vi "Last Ack.vi"(7 "Sender":refnum<class "Sender.lvclass">, 10 "Actor":refnum<class "Actor.lvclass">, 11 "jettl Actor in":refnum<class "jettl Actor.lvclass">) -> (3 "jettl Actor out":refnum<class "jettl Actor.lvclass">)   [LabVIEW 2021, in "jettl.lvlib" / "Temporary Actor.lvlib" / "jettl Actor.lvclass"]
uses:
  jettl Actor.lvclass
  Actor/Actor.lvclass
  Sender/Sender/Sender.lvclass
  jettl Actor.lvclass/jettl Actor.ctl
  Addresses Strategy/Addresses Strategy/Addresses Strategy.lvclass
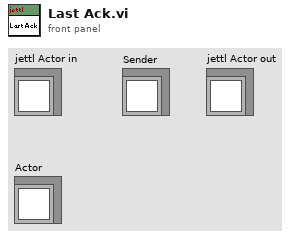
[diagram p1: front panel]
types:
  T1 = typedef "jettl.lvlib/Relation.ctl" = enum16{"Self", "Creator", "Created"}
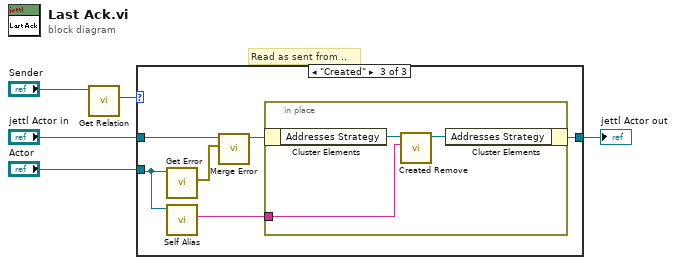
[diagram p0: block diagram]
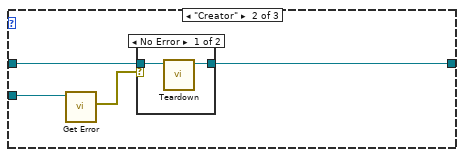
[diagram p3: hidden frame]
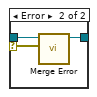
[diagram p4: hidden frame]
diagram:
  # "Read as sent from .."
  n1 = call-dynamic "Get Relation.vi"("Sender in"="Sender") -> ("Relation"=w1:T1)  [unwired: 10 in]
  n2 = case shown="\"Created\"" w1 {
    tunnel: "jettl Actor in" -> [w6 w9 w18]
    tunnel: [w6 w8 w17] -> w4
    tunnel: "Actor" -> [_ w7 w16]
    frame "Self" {
      # "Case will not fundamentally exist"
    }
    frame "Creator" {
      n3 = call-dynamic "Get Error.vi"("Actor in"=w7) -> ("Error"=w10:errorcluster)  [unwired: 10 in]
      n4 = case shown="No Error" w10 {
        selector: w10 -> [_ w15]
        tunnel: w9 -> [w12 w14]
        tunnel: [w11 w13] -> w8
        frame No Error {
          n5 = call-dynamic "Teardown.vi"("jettl Actor in"=w12) -> ("jettl Actor out"=w11:refnum<class "jettl Actor.lvclass">)  [unwired: 10 in]
        }
        frame Error {
          n6 = call-dynamic "Merge Error.vi"("Error"=w15, "jettl Actor in"=w14) -> ("jettl Actor out"=w13:refnum<class "jettl Actor.lvclass">)  [unwired: 9 in]
        }
      }
    }
    frame "Created" {
      n7 = call-dynamic "Get Error.vi"("Actor in"=w16) -> ("Error"=w21:errorcluster)  [unwired: 10 in]
      n8 = call-dynamic "Self Alias.vi"("Actor in"=w16) -> ("Self Alias"=w20:string)  [unwired: 10 in]
      n9 = call-dynamic "Merge Error.vi"("Error"=w21, "jettl Actor in"=w18) -> ("jettl Actor out"=w19:refnum<class "jettl Actor.lvclass">)  [unwired: 9 in]
      n10 = in-place {
        in-place-border: w20 -> [w22]
        n11 = in-place-cluster #1(w19) -> ("Addresses Strategy"=w24:refnum<class "Addresses Strategy.lvclass">)
        n12 = call-dynamic "Created Remove.vi"("Created Alias"=w22, "Addresses Strategy in"=w24) -> ("Addresses Strategy out"=w23:refnum<class "Addresses Strategy.lvclass">)  [unwired: 9 in]
        n13 = in-place-cluster #1("Addresses Strategy"=w23) -> (w17:refnum<class "jettl Actor.lvclass">)
      }
    }
  }
  "jettl Actor out" <- w4
